vi "MainInterface.vi"() -> ()   [LabVIEW 2014]
uses:
  globe stop.vi
  DistGlobal.vi
  <vilib>/imath/engines/lvmath2/RunTimeEngine/Managers/WorkSpace/UID Generator.vi
  <vilib>/imath/engines/lvmath2/RunTimeEngine/RangeToken/NIMS_Range.vi
  <instcachedir>/0/NIMS_Range_9BCE657718DF4976A877346C61F22738.lvgen/NIMS_Range_9BCE657718DF4976A877346C61F22738_000.vi
  <vilib>/imath/engines/lvmath2/RunTimeEngine/RunTimeType/NIMS_RunTimeType_From StrictType (excl LVString).vi
  <instcachedir>/0/NIMS_RunTimeType_From StrictType (excl LVString)_15A5391EEA9C4AACB9955AC755B83D29.lvgen/NIMS_RunTimeType_From StrictType (excl LVString)_15A5391EEA9C4AACB9955AC755B83D29_000.vi
  <vilib>/imathl/engines/lvmath/Functions/Error Handling/Create Error.vi
  <vilib>/imath/engines/lvmath2/RunTimeEngine/LocalVariableDefStatement/MC_LocalVariableDefStatement_Display.vi
  <vilib>/imath/engines/lvmath2/RunTimeEngine/RangeToken/NIMS_Range_R3 - Integer.vi
  <instcachedir>/0/NIMS_Range_R3 - Integer_66B9031982364693905FDE422E56E490.lvgen/NIMS_Range_R3 - Integer_66B9031982364693905FDE422E56E490_000.vi
  <vilib>/imath/engines/lvmath2/RunTimeEngine/CommandStatement/MC_CommandStatement_break.vi
  <vilib>/imath/engines/lvmath2/RunTimeEngine/Managers/SymbolTable/Clear UID.vi
  <vilib>/imath/engines/lvmath2/RunTimeEngine/NodeEndStatement/NIMS_NodeEndStatement_Output.vi
  <instcachedir>/0/NIMS_NodeEndStatement_Output_53EC0D466D134D7ABD903AC30B43404B.lvgen/NIMS_NodeEndStatement_Output_53EC0D466D134D7ABD903AC30B43404B_005.vi
  <vilib>/imath/engines/lvmath2/RunTimeEngine/ErrorHandling/NIMS_Finalize Error.vi
  StepperData.vi
  <instcachedir>/0/NIMS_NodeEndStatement_Output_53EC0D466D134D7ABD903AC30B43404B.lvgen/NIMS_NodeEndStatement_Output_53EC0D466D134D7ABD903AC30B43404B_001.vi
  <vilib>/imath/engines/lvmath2/RunTimeEngine/Managers/SymbolTable/NIMS_WorkSpace.lvlib
panel:
  in  "Echo Term":tag="Dev1/ctr1"
  in  "Trigger Term":tag="Dev1/ctr0"
  in  "Speed (int 1 to 10)":i32
  in  "Sweep Angle\n(9 degree increments work best)":i32
  out "Range":cluster{"Y":dbl[], "Y":dbl[]}[](graph)
  in  "?":bool
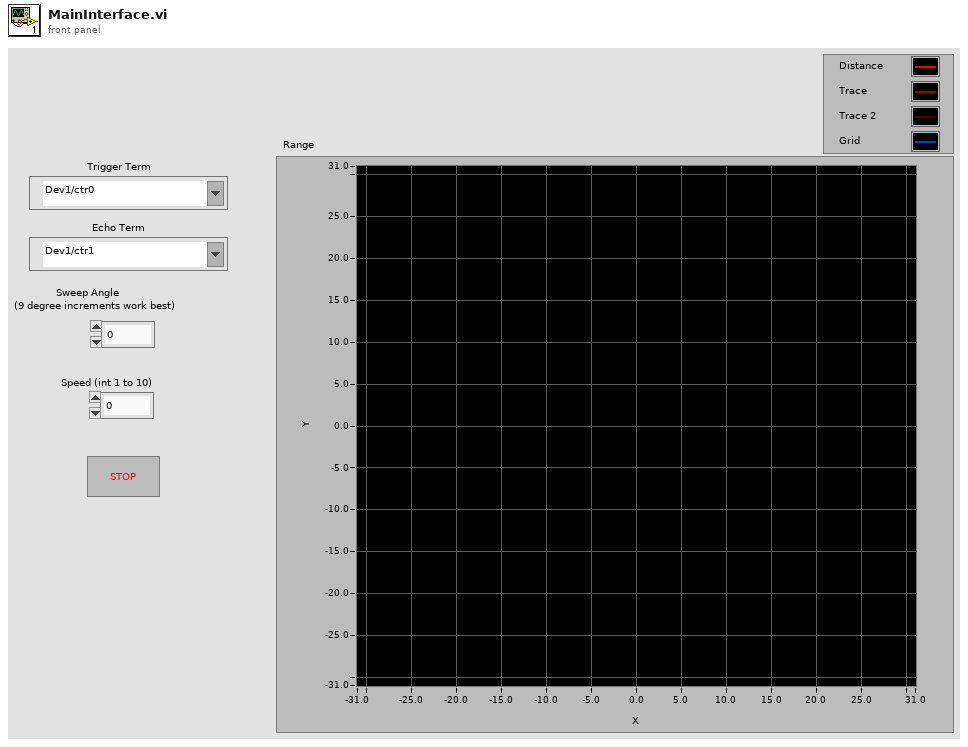
[diagram p1: front panel]
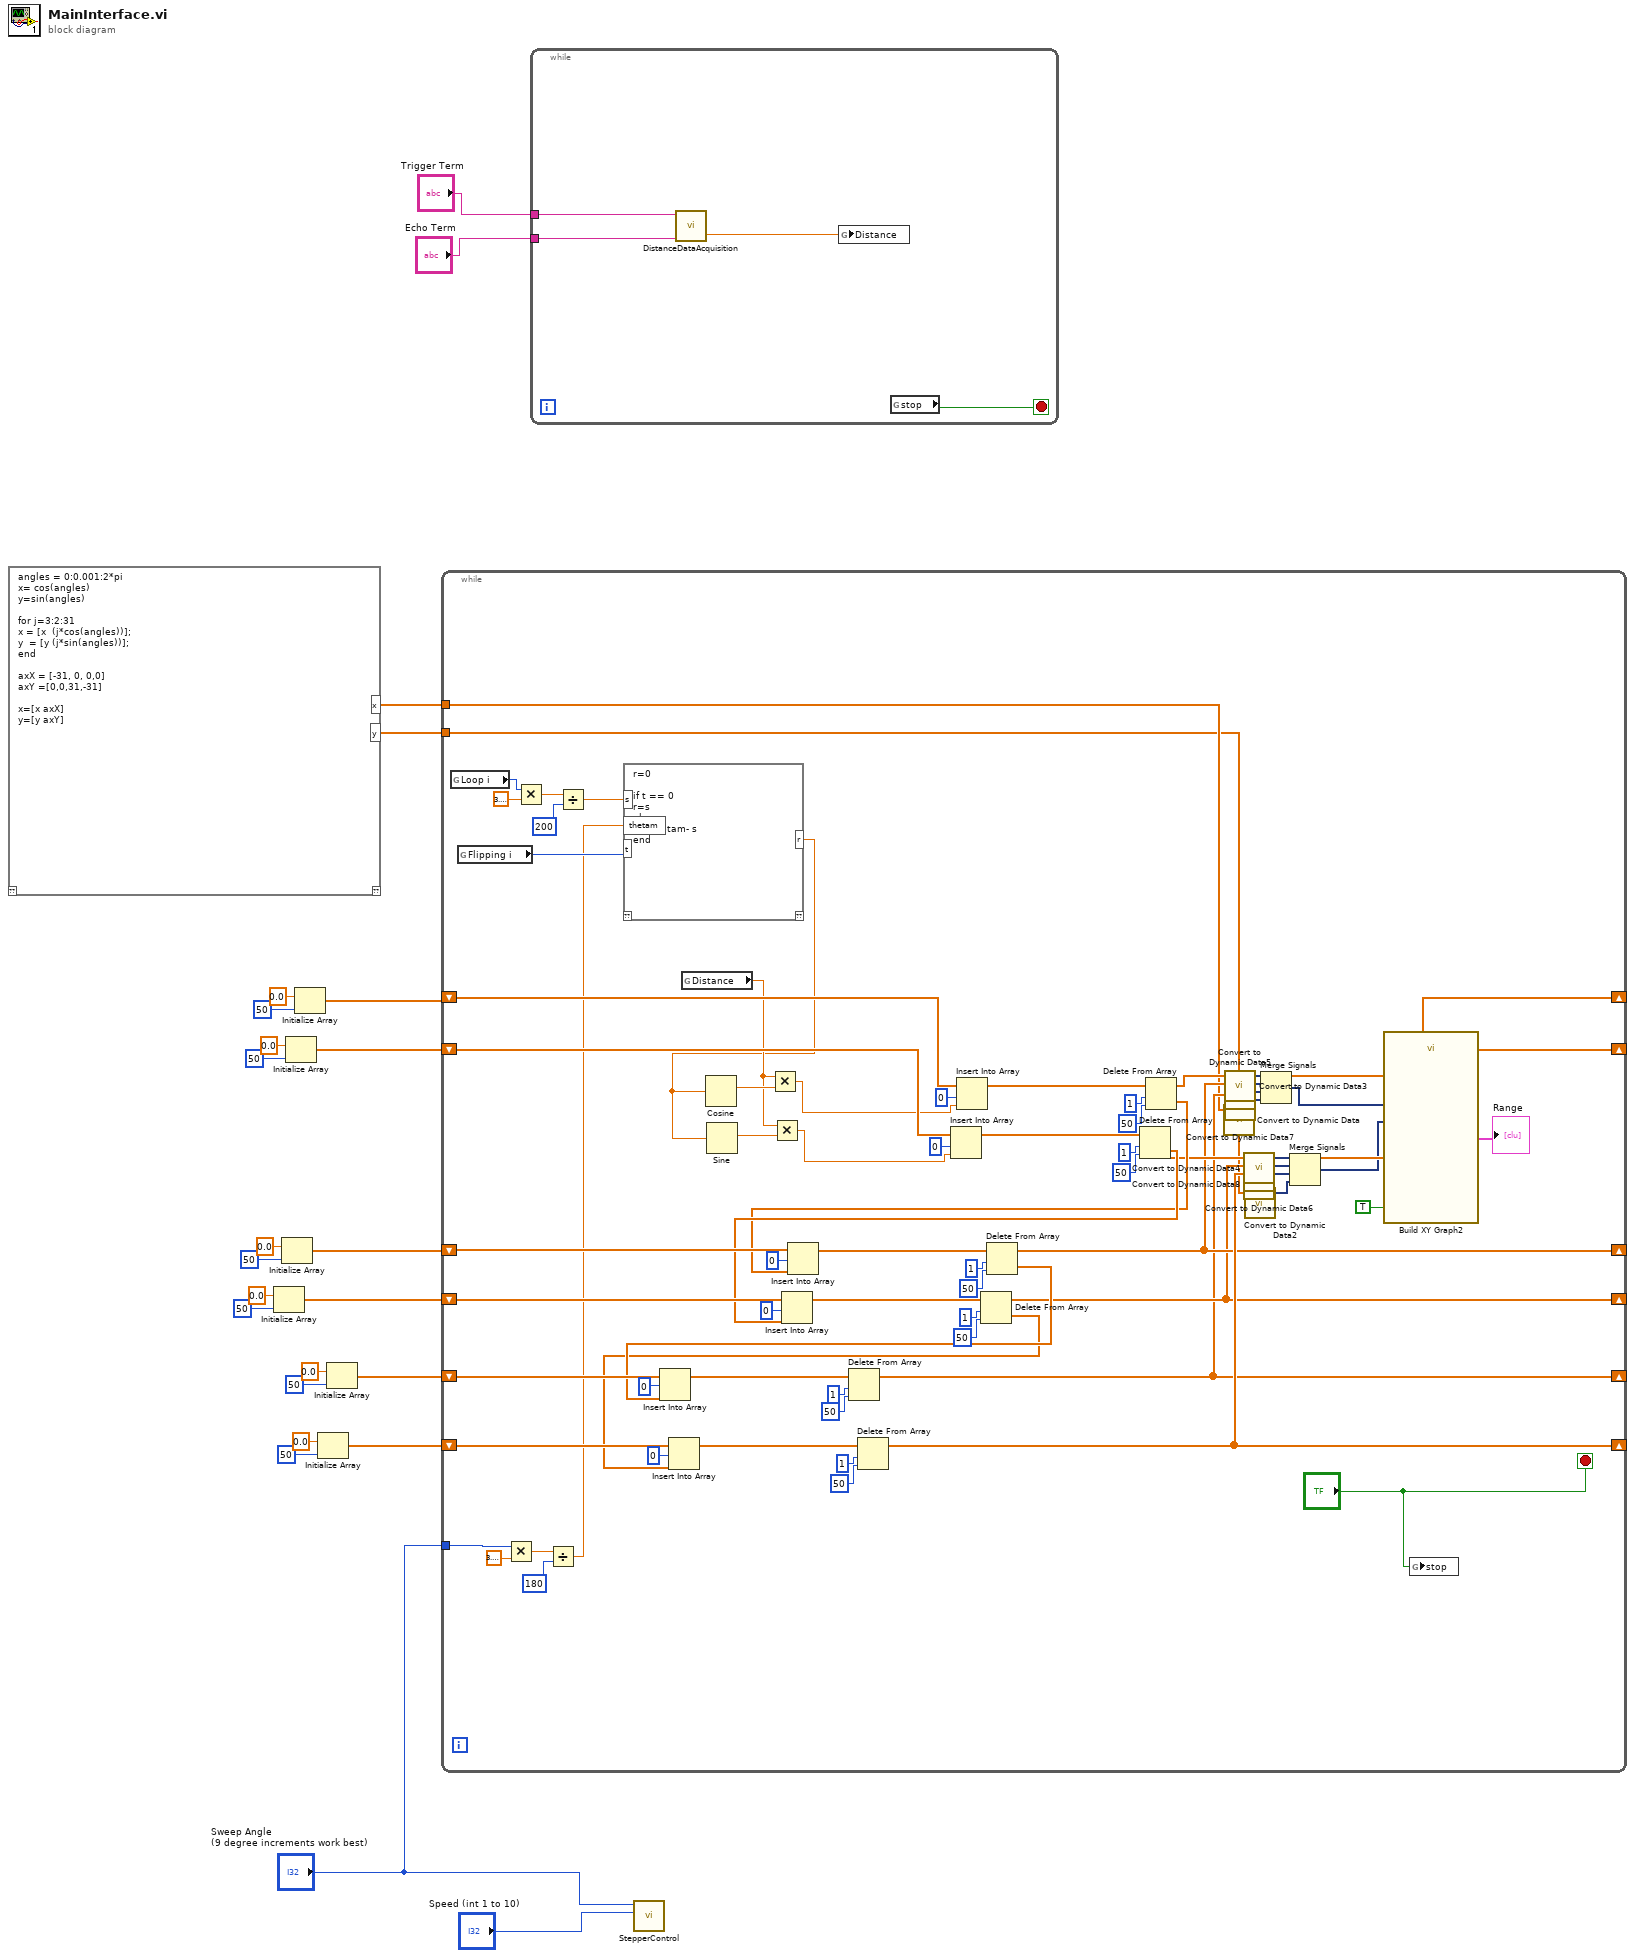
[diagram p0: block diagram]
diagram:
  n1 = mathscript code="angles = 0:0.001:2*pi\nx= cos(angles)\ny=sin(angles)\n\nfor j=3:2:31\nx = [x  (j*cos(angles))];\ny  = [y (j*sin(angles))];\nend\n\naxX = [-31, 0, 0,0]\naxY =[0,0,31,-31]\n\nx=[x axX]\ny=[y axY]"() -> ("x"=w6:dbl[], "y"=w5:dbl[])  [unwired: 1 in, 1 out]
  n2 = Initialize Array(0.0 ("element"), 50 ("dimension size")) -> (w9:dbl[])
  n3 = Initialize Array(0.0 ("element"), 50 ("dimension size")) -> (w10:dbl[])
  n4 = Initialize Array(0.0 ("element"), 50 ("dimension size")) -> (w8:dbl[])
  n5 = Initialize Array(0.0 ("element"), 50 ("dimension size")) -> (w7:dbl[])
  n6 = Initialize Array(0.0 ("element"), 50 ("dimension size")) -> (w22:dbl[])
  n7 = Initialize Array(0.0 ("element"), 50 ("dimension size")) -> (w19:dbl[])
  n8 = while {
    shift-right: [w43] -> _
    shift-left: w9 -> [w63]
    shift-right: [w44] -> _
    shift-left: w10 -> [w62]
    shift-right: [w48] -> _
    shift-left: w22 -> [w89]
    shift-right: [w42] -> _
    shift-left: w19 -> [w64]
    shift-right: [w46] -> _
    shift-left: w7 -> [w60]
    shift-right: [w45] -> _
    shift-left: w8 -> [w61]
    tunnel: w6 -> [w37]
    tunnel: w5 -> [w26]
    tunnel: "Sweep Angle\n(9 degree increments work best)" -> [w28]
    stop <- "?" stop-if-true
    n9 = global read "StepperData.vi" "Loop i"() -> (w33:i32)
    n10 = global read "StepperData.vi" "Flipping i"() -> (w34:i32)
    n11 = Multiply(x=w28, y=3.141592653589793) -> (x*y=w31:dbl)
    n12 = Multiply(x=w33, y=3.141592653589793) -> (x*y=w92:dbl)
    n13 = Divide(x=w31, y=180) -> (x/y=w27:dbl)
    n14 = Divide(x=w92, y=200) -> (x/y=w32:dbl)
    n15 = mathscript code="r=0\n\nif t == 0\nr=s\nelse\nr = thetam- s\nend"("s"=w32, "t"=w34, "thetam"=w27) -> ("r"=w35:dbl)  [unwired: 1 in, 1 out]
    n16 = global read "DistGlobal.vi" "Distance"() -> (w36:dbl)
    n17 = Cosine(x=w35) -> (cos(x)=w90:dbl)
    n18 = Sine(x=w35) -> (sin(x)=w95:dbl)
    n19 = Multiply(x=w36, y=w90) -> (x*y=w59:dbl)
    n20 = Multiply(x=w36, y=w95) -> (x*y=w58:dbl)
    n21 = Insert Into Array(array=w61, index=0, new element=w58) -> (w69:dbl[])
    n22 = Insert Into Array(array=w60, index=0, new element=w59) -> (w68:dbl[])
    n23 = Delete From Array(array=w69, length=1, index=50) -> (deleted portion=w57:dbl[], array with subset deleted=w45:dbl[])
    n24 = Insert Into Array(array=w63, index=0, new element=w57) -> (w76:dbl[])
    n25 = Delete From Array(array=w76, length=1, index=50) -> (deleted portion=w54:dbl[], array with subset deleted=w43:dbl[])
    n26 = Insert Into Array(array=w89, index=0, new element=w54) -> (w85:dbl[])
    n27 = Delete From Array(array=w85, length=1, index=50) -> (array with subset deleted=w48:dbl[])  [unwired: 1 out]
    n28 = Delete From Array(array=w68, length=1, index=50) -> (deleted portion=w56:dbl[], array with subset deleted=w46:dbl[])
    n29 = Insert Into Array(array=w62, index=0, new element=w56) -> (w77:dbl[])
    n30 = Delete From Array(array=w77, length=1, index=50) -> (deleted portion=w55:dbl[], array with subset deleted=w44:dbl[])
    n31 = Insert Into Array(array=w64, index=0, new element=w55) -> (w84:dbl[])
    n32 = Delete From Array(array=w84, length=1, index=50) -> (array with subset deleted=w42:dbl[])  [unwired: 1 out]
    n33 = call "Convert to Dynamic Data"("Array"=w37) -> ("Dynamic Data Type"=w41:dynamicdata)  [unwired: 3 in]
    n34 = call "Convert to Dynamic Data3"("Array"=w46) -> ("Dynamic Data Type"=w53:dynamicdata)  [unwired: 3 in]
    n35 = call "Convert to Dynamic Data5"("Array"=w44) -> ("Dynamic Data Type"=w51:dynamicdata)  [unwired: 3 in]
    n36 = call "Convert to Dynamic Data7"("Array"=w42) -> ("Dynamic Data Type"=w49:dynamicdata)  [unwired: 3 in]
    n37 = call "Convert to Dynamic Data4"("Array"=w45) -> ("Dynamic Data Type"=w52:dynamicdata)  [unwired: 3 in]
    n38 = call "Convert to Dynamic Data6"("Array"=w43) -> ("Dynamic Data Type"=w50:dynamicdata)  [unwired: 3 in]
    n39 = call "Convert to Dynamic Data8"("Array"=w48) -> ("Dynamic Data Type"=w47:dynamicdata)  [unwired: 3 in]
    n40 = call "Convert to Dynamic Data2"("Array"=w26) -> ("Dynamic Data Type"=w40:dynamicdata)  [unwired: 3 in]
    n41 = Merge Signals(w53, w51, w49, w41) -> (w39:dynamicdata)
    n42 = Merge Signals(w52, w50, w47, w40) -> (w38:dynamicdata)
    n43 = call "Build XY Graph2"("Reset"=TRUE, "Y Input"=w38, "X Input"=w39) -> ("XY Graph"=→"Range":cluster{"X":dbl[], "Y":dbl[]}[])  [unwired: 7 in, 1 out]
    n44 = global write "globe stop.vi" "stop"("?") -> ()
  }
  n45 = while {
    tunnel: "Trigger Term" -> [w179]
    tunnel: "Echo Term" -> [w178]
    stop <- w180 stop-if-true
    n46 = call "DistanceDataAcquisition.vi"("Echo Term"=w178, "Trigger Term"=w179) -> ("Distance (IN)"=w181:dbl)  [unwired: 9 in]
    n47 = global write "DistGlobal.vi" "Distance"(w181) -> ()
    n48 = global read "globe stop.vi" "stop"() -> (w180:bool)
  }
  n49 = call "StepperControl.vi"("speed"="Speed (int 1 to 10)", "sweep angle\n(9 degree increments work best)"="Sweep Angle\n(9 degree increments work best)") -> ()  [unwired: 10 in]
